vi "scanner_v2 Josh Oborn (possible camera fix).vi"() -> ()   [LabVIEW 2020]
uses:
  C:/Program Files/Thorlabs/Scientific Imaging/DCx Camera Support/Develop/DotNet/uc480DotNet.dll
  Program Files/Thorlabs/Scientific Imaging/DCx Camera Support/Develop/DotNet/uc480DotNet.dll
  System.Windows.Forms
panel:
  in  "Rotation Stage Motor":refnum<k7>(container)
  in  "Mode":i32(ring) items=["BGRA8Packed"=0, "BGR8Packed"=1, "BGR565Packed"=2, "BGR5Packed"=3, "Mono8"=6, "SensorRaw8"=11, "UYVYPacked"=12, "UYVYMonoPacked"=13, "UYVYBayerPacked"=14, "CBYCRYPacked"=23, "BGRY8Packed"=24, "BGR10Packed"=25, "Mono12"=26, "SensorRaw12"=27, "Mono16"=28, "SensorRaw16"=29, "BGR12Unpacked"=30, "BGRA12Unpacked"=31, "Jpeg"=32, "SensorRaw10"=33, "Mono10"=34, "BGR10Unpacked"=35, "RGBA8Packed"=128, "RGB8Packed"=129, "RGBY8Packed"=152, "RGB10Packed"=153, "RGB12Unpacked"=158, "RGBA12Unpacked"=159, "RGB10Unpacked"=163, "RGB8Planar"=8321, "PreferPackedSourceFormat"=16384]
  in  "Picture Box":refnum<k24>(container)
  in  "?":bool
  out "Total Translation":sgl
  out "fAbsPosCh2":sgl
  in  "Translation Stage Motor":refnum<k7>(container)
  in  "Number Of Translation Steps":i32=100
  out "error out":errorcluster
  in  "Number Of Rotation Steps":i32=100
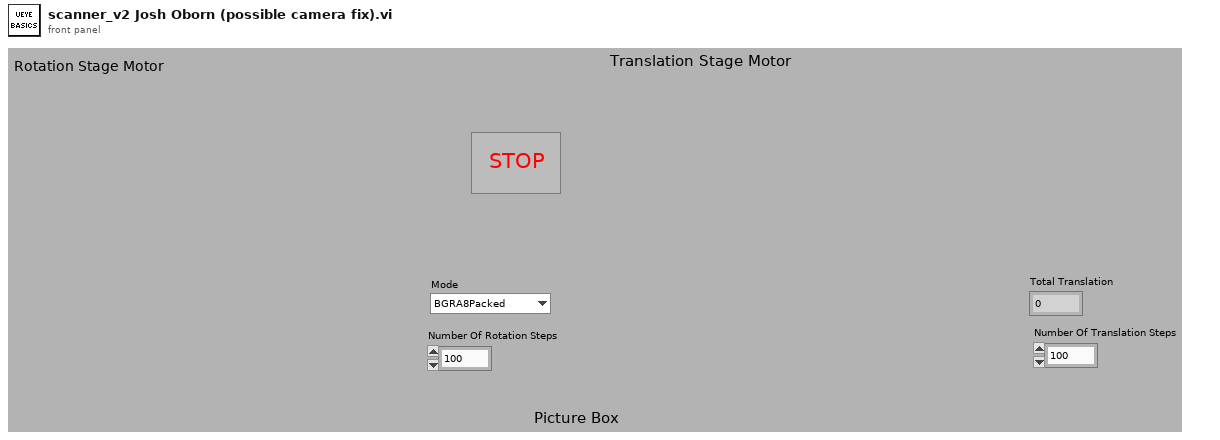
[diagram p1: front panel]
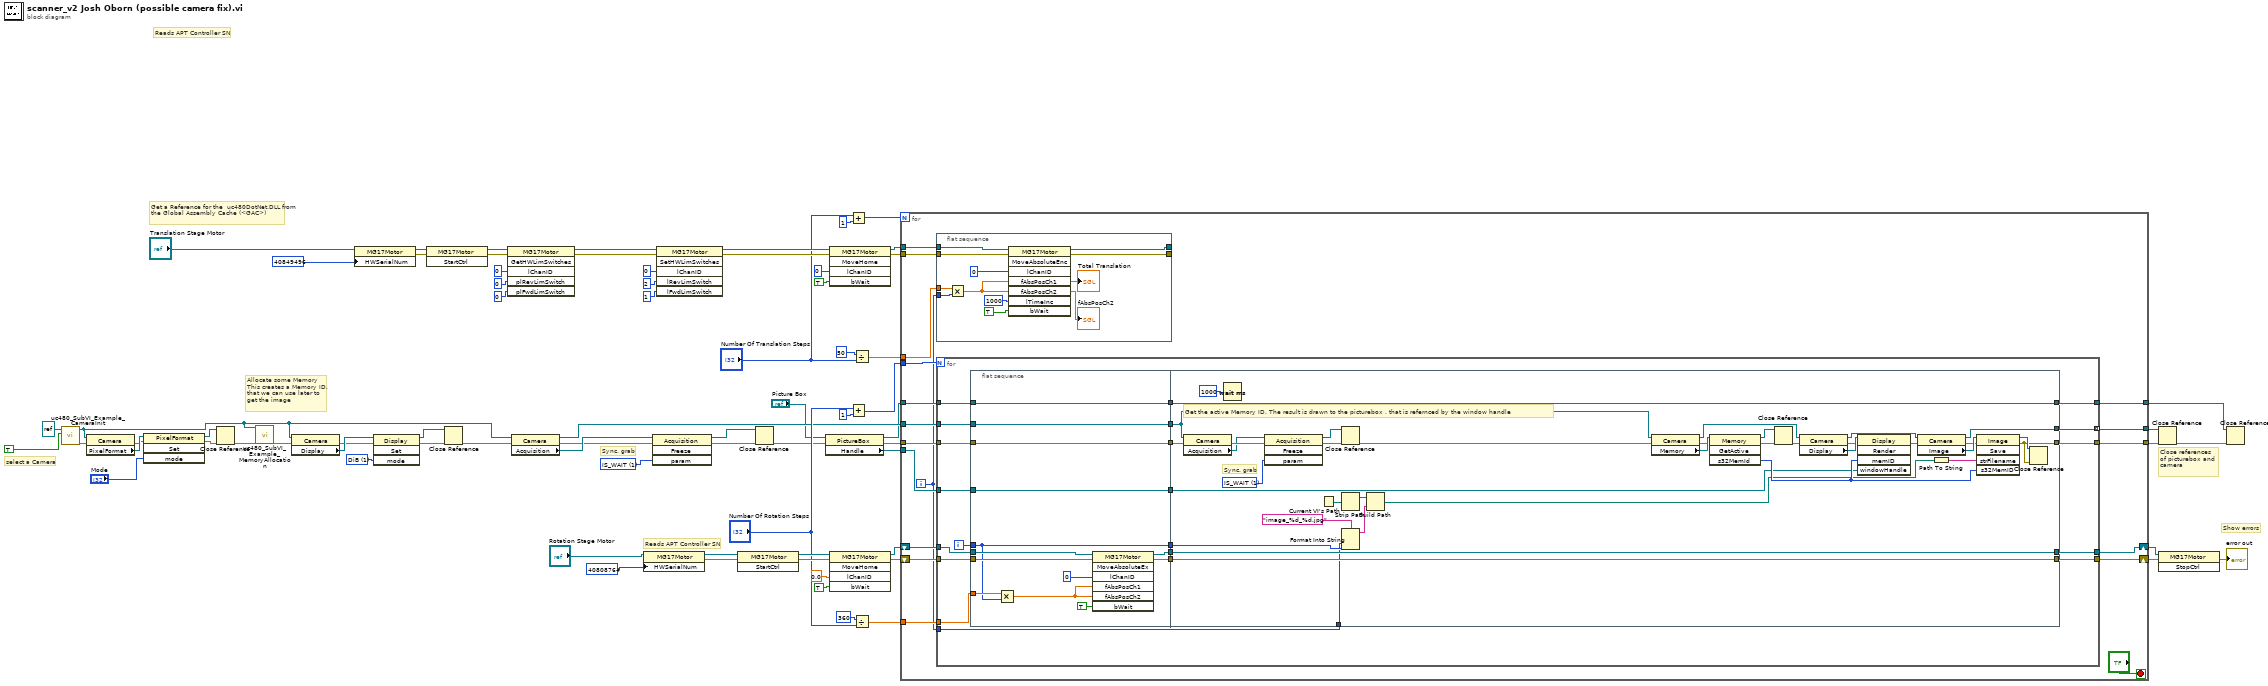
[diagram p0: block diagram]
diagram:
  w59 = 1 items=["DiB"=1, "Direct3D"=4, "OpenGL"=8, "Mono"=2048, "Bayer"=4096] ("mode")
  w72 = 1 items=["IS_DONT_WAIT", "IS_WAIT"] ("Wait")
  # "Reads APT Controller SN"
  # "Reads APT Controller SN"
  # "Close references\nof picturebox and camera"
  # "Show errors"
  # "Allocate some Memory\nThis creates a Memory ID,\nthat we can use later to\nget the image"
  # "Sync. grab"
  # "select a Camera"
  # "Get a Reference for the  uc480DotNet.DLL from the Global Assembly Cache (<GAC>)"
  n1 = call "uc480_SubVI_Example_CameraInit.vi"("Init Camera Flag"=TRUE ("Init Camera"), ".NET (Reference)"=refnum<k24> refnum (".NET (Referenz)")) -> ("Error Out"=w69:errorcluster, ".NET (Reference)"=w54:refnum<k24>)  [unwired: 8 in]
  n2 = property class="Camera"(reference=w54, error in=w69) -> (error out=w70:errorcluster, "PixelFormat"=w71:refnum<k24>)  [unwired: 1 out]
  n3 = invoke class="PixelFormat" method="Set"(reference=w71, error in=w70, "mode"="Mode") -> (reference out=w68:refnum<k24>, error out=w67:errorcluster)  [unwired: 1 in, 2 out]
  n4 = Close Reference(reference=w68, error in (no error)=w67) -> (error out=w66:errorcluster)
  n5 = call "uc480_SubVI_Example_MemoryAllocation.vi"(".NET (Reference)"=w54, "Error In"=w66) -> ("Error Out"=w61:errorcluster)  [unwired: 13 in, 4 out]
  n6 = property class="Camera"(reference=w54, error in=w61) -> (error out=w58:errorcluster, "Display"=w60:refnum<k24>)  [unwired: 1 out]
  n7 = property class="MG17Motor"(reference="Translation Stage Motor", "HWSerialNum"=40849496) -> (reference out=w26:refnum<k7>, error out=w25:errorcluster)  [unwired: 1 in]
  n8 = invoke class="Display" method="Set"(reference=w60, error in=w58, "mode"=w59) -> (reference out=w57:refnum<k24>, error out=w56:errorcluster)  [unwired: 1 in, 2 out]
  n9 = invoke class="MG17Motor" method="StartCtrl"(reference=w26, error in=w25) -> (reference out=w24:refnum<k7>, error out=w23:errorcluster)  [unwired: 1 in, 1 out]
  n10 = Close Reference(reference=w57, error in (no error)=w56) -> (error out=w55:errorcluster)
  n11 = invoke class="MG17Motor" method="GetHWLimSwitches"(reference=w24, error in=w23, "lChanID"=0, "plRevLimSwitch"=0, "plFwdLimSwitch"=0) -> (reference out=w12:refnum<k7>, error out=w13:errorcluster)  [unwired: 1 in, 4 out]
  n12 = property class="Camera"(reference=w54, error in=w55) -> (reference out=w43:refnum<k24>, error out=w73:errorcluster, "Acquisition"=w74:refnum<k24>)
  n13 = property class="MG17Motor"(reference="Rotation Stage Motor", "HWSerialNum"=40808764) -> (reference out=w53:refnum<k7>, error out=w52:errorcluster)  [unwired: 1 in]
  n14 = invoke class="Acquisition" method="Freeze"(reference=w74, error in=w73, "param"=w72) -> (reference out=w64:refnum<k24>, error out=w65:errorcluster)  [unwired: 1 in, 2 out]
  n15 = invoke class="MG17Motor" method="SetHWLimSwitches"(reference=w12, error in=w13, "lChanID"=0, "lRevLimSwitch"=2 ("plRevLimSwitch"), "lFwdLimSwitch"=1 ("plFwdLimSwitch")) -> (reference out=w15:refnum<k7>, error out=w14:errorcluster)  [unwired: 1 in, 4 out]
  n16 = invoke class="MG17Motor" method="StartCtrl"(reference=w53, error in=w52) -> (reference out=w50:refnum<k7>, error out=w51:errorcluster)  [unwired: 1 in, 1 out]
  n17 = Close Reference(reference=w64, error in (no error)=w65) -> (error out=w35:errorcluster)
  n18 = property class="PictureBox"(reference="Picture Box", error in=w35) -> (reference out=w32:refnum<k24>, error out=w34:errorcluster, "Handle"=w33:refnum<k24>)
  n19 = invoke class="MG17Motor" method="MoveHome"(reference=w15, error in=w14, "lChanID"=0, "bWait"=TRUE) -> (reference out=w6:refnum<k7>, error out=w7:errorcluster)  [unwired: 1 in, 3 out]
  n20 = invoke class="MG17Motor" method="MoveHome"(reference=w50, error in=w51, "lChanID"=0.0, "bWait"=TRUE) -> (reference out=w40:refnum<k7>, error out=w41:errorcluster)  [unwired: 1 in, 3 out]
  n21 = Add(x="Number Of Translation Steps", y=1) -> (x+y=w28:i32)
  n22 = Add(x="Number Of Rotation Steps", y=1) -> (x+y=w44:i32)
  n23 = Divide(x=50, y="Number Of Translation Steps") -> (x/y=w8:dbl)
  n24 = Divide(x=360, y="Number Of Rotation Steps") -> (x/y=w36:dbl)
  n25 = for {
    N: w28 -> [_]
    tunnel: w44 -> [w93]
    tunnel: w43 -> [w92]
    tunnel: [w91] -> w42
    tunnel: w36 -> [w86]
    shift-right: [w87] -> w37
    shift-left: w41 -> [w90]
    shift-right: [w88] -> w38
    shift-left: w40 -> [w89]
    tunnel: w34 -> [w85]
    tunnel: w33 -> [w84]
    tunnel: w32 -> [w83]
    tunnel: [w82] -> w31
    tunnel: [w81] -> w30
    tunnel: w8 -> [w80]
    tunnel: w7 -> [w79]
    tunnel: w6 -> [w78]
    i -> [w76]
    stop <- "?" stop-if-true
    n26 = flat-sequence {
      tunnel: w78 -> [w104]
      tunnel: w79 -> [w103]
      tunnel: w76 -> [w100]
      tunnel: w80 -> [w99]
      tunnel: [w102] -> _
      tunnel: [w101] -> _
      frame #0 {
        n27 = Multiply(x=w99, y=w100) -> (x*y=w97:dbl)
        n28 = invoke class="MG17Motor" method="MoveAbsoluteEnc"(reference=w104, error in=w103, "lChanID"=0, "fAbsPosCh1"=w97, "fAbsPosCh2"=w97, "lTimeInc"=1000, "bWait"=TRUE) -> (reference out=w102:refnum<k7>, error out=w101:errorcluster, "fAbsPosCh1"=→"Total Translation":sgl, "fAbsPosCh2"=→"fAbsPosCh2":sgl)  [unwired: 1 in, 4 out]
      }
    }
    n29 = for {
      N: w93 -> [_]
      tunnel: w85 -> [w124]
      tunnel: w92 -> [w125]
      tunnel: w84 -> [w123]
      tunnel: [w118] -> w82
      tunnel: w83 -> [w126]
      tunnel: [w117] -> w81
      tunnel: [w116] -> w91 mode=indexing
      tunnel: w90 -> [w115]
      tunnel: w89 -> [w114]
      tunnel: [w111] -> w88
      tunnel: [w110] -> w87
      tunnel: w86 -> [w109]
      tunnel: w76 -> [w106]
      i -> [w108]
      n30 = flat-sequence {
        tunnel: w126 -> [w139]
        tunnel: w125 -> [w138]
        tunnel: w124 -> [w137]
        tunnel: w123 -> [w136]
        tunnel: [w139] -> w122
        tunnel: [w138] -> w121
        tunnel: [w137] -> w120
        tunnel: [w136] -> w119
        tunnel: w115 -> [w132]
        tunnel: w114 -> [w131]
        tunnel: [w130] -> w113
        tunnel: [w129] -> w112
        tunnel: w109 -> [w128]
        tunnel: w108 -> [w127]
        tunnel: [w127] -> w107
        tunnel: [w149] -> w118
        tunnel: w122 -> [w149]
        tunnel: w121 -> [w147]
        tunnel: w120 -> [w148]
        tunnel: w119 -> [w146]
        tunnel: [w145] -> w117
        tunnel: [w144] -> w116
        tunnel: w113 -> [w142]
        tunnel: w112 -> [w143]
        tunnel: [w143] -> w111
        tunnel: [w142] -> w110
        tunnel: w107 -> [w141]
        tunnel: w106 -> [w140]
        frame #0 {
          n31 = Multiply(x=w128, y=w127) -> (x*y=w135:dbl)
          n32 = invoke class="MG17Motor" method="MoveAbsoluteEx"(reference=w131, error in=w132, "lChanID"=0, "fAbsPosCh1"=w135, "fAbsPosCh2"=w135, "bWait"=TRUE) -> (reference out=w129:refnum<k7>, error out=w130:errorcluster)  [unwired: 1 in, 5 out]
        }
        frame #1 {
          w163 = 1 items=["IS_DONT_WAIT", "IS_WAIT"] ("Wait")
          # "Sync. grab"
          # "Get the active Memory ID. The result is drawn to the picturebox , that is refernced by the window handle"
          n33 = property class="Camera"(reference=w147, error in=w148) -> (error out=w165:errorcluster, "Acquisition"=w164:refnum<k24>)  [unwired: 1 out]
          n34 = Wait (ms)(milliseconds to wait=u32 1000) -> ()  [unwired: 1 out]
          n35 = invoke class="Acquisition" method="Freeze"(reference=w164, error in=w165, "param"=w163) -> (reference out=w167:refnum<k24>, error out=w166:errorcluster)  [unwired: 1 in, 2 out]
          n36 = Current VI's Path() -> (path=w155:path)
          n37 = Close Reference(reference=w167, error in (no error)=w166) -> (error out=w162:errorcluster)
          n38 = Strip Path(path=w155) -> (stripped path=w154:path)  [unwired: 1 out]
          n39 = Format Into String(format string="image_%d_%d.jpg", w140, w141) -> (resulting string=w151:string)  [unwired: 2 in, 1 out]
          n40 = Build Path(base path=w154, name or relative path=w151) -> (appended path=w153:path)
          n41 = property class="Camera"(reference=w147, error in=w162) -> (reference out=w169:refnum<k24>, error out=w175:errorcluster, "Memory"=w176:refnum<k24>)
          n42 = invoke class="Memory" method="GetActive"(reference=w176, error in=w175) -> (reference out=w173:refnum<k24>, error out=w172:errorcluster, "s32MemId"=w159:i32)  [unwired: 2 in, 1 out]
          n43 = Close Reference(reference=w173, error in (no error)=w172) -> (error out=w171:errorcluster)
          n44 = property class="Camera"(reference=w169, error in=w171) -> (reference out=w161:refnum<k24>, error out=w170:errorcluster, "Display"=w174:refnum<k24>)
          n45 = invoke class="Display" method="Render"(reference=w174, error in=w170, "memID"=w159, "windowHandle"=w146) -> (error out=w158:errorcluster)  [unwired: 1 in, 4 out]
          n46 = property class="Camera"(reference=w161, error in=w158) -> (reference out=w144:refnum<k24>, error out=w157:errorcluster, "Image"=w160:refnum<k24>)
          n47 = Path To String(path=w153) -> (string=w152:string)
          n48 = invoke class="Image" method="Save"(reference=w160, error in=w157, "strFilename"=w152, "s32MemID"=w159) -> (reference out=w156:refnum<k24>, error out=w145:errorcluster)  [unwired: 1 in, 3 out]
          n49 = Close Reference(reference=w156, error in (no error)=w145) -> ()  [unwired: 1 out]
        }
      }
    }
  }
  n50 = invoke class="MG17Motor" method="StopCtrl"(reference=w38, error in=w37) -> (error out=→"error out":errorcluster)  [unwired: 1 in, 2 out]
  n51 = Close Reference(reference=w42, error in (no error)=w30) -> (error out=w63:errorcluster)
  n52 = Close Reference(reference=w31, error in (no error)=w63) -> ()  [unwired: 1 out]
